vi "Update distance annotations.vi"(5 "Y axis max":dbl, 7 "Y axis min":dbl, 8 "error in (no error)":errorcluster, 9 "Anott. for update array in":i32[](array[numeric]), 10 "All cursors' dist.":T2, 11 "XY Graph":refnum<vi>) -> (0 "error out":errorcluster)   [LabVIEW 2014]
uses:
  Controls/dist. between cursors.ctl
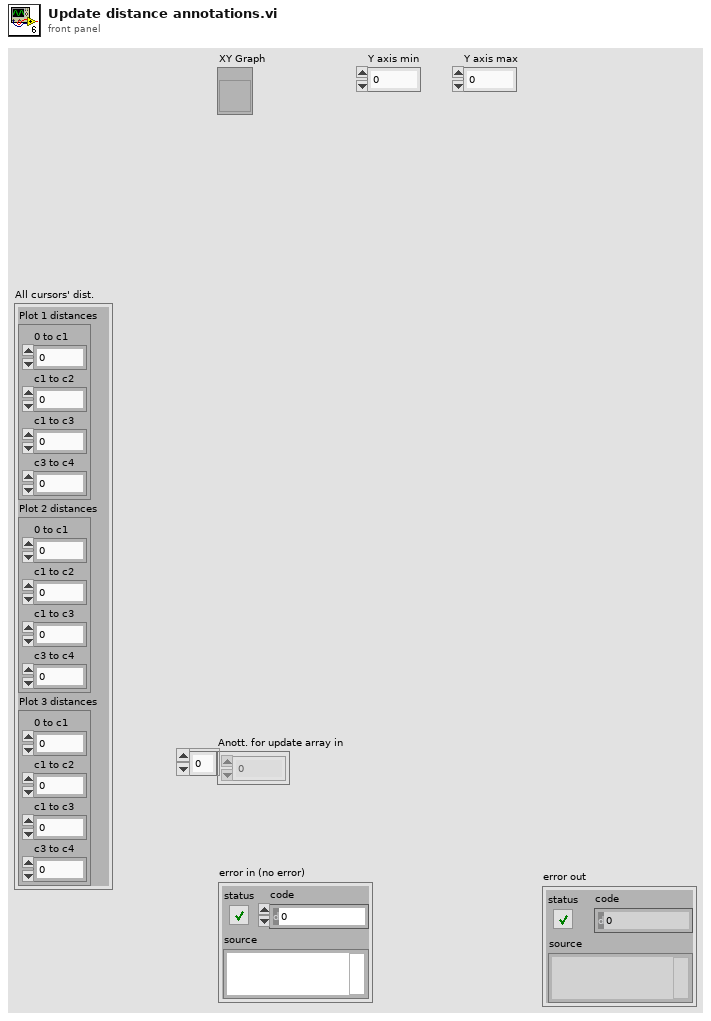
[diagram p1: front panel]
types:
  T1 = typedef "dist. between cursors.ctl" = cluster{"0 to c1":dbl, "c1 to c2":dbl, "c1 to c3":dbl, "c3 to c4":dbl}
  T2 = cluster{"Plot 1 distances":T1, "Plot 2 distances":T1, "Plot 3 distances":T1}
  T3 = enum16{"read", "write", "write number of cursors per plot only"}
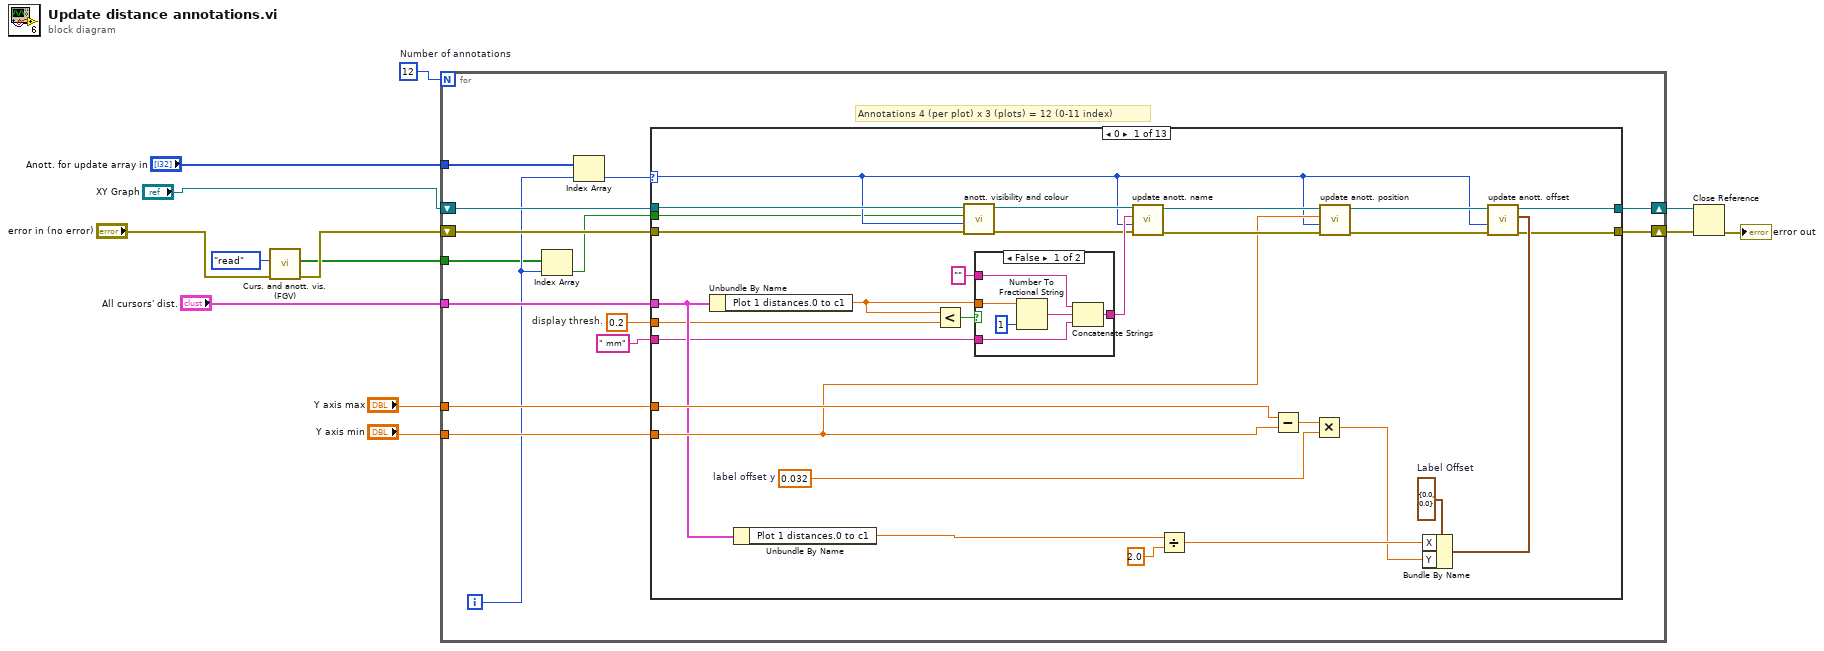
[diagram p0: block diagram]
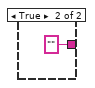
[diagram p2: hidden frame]
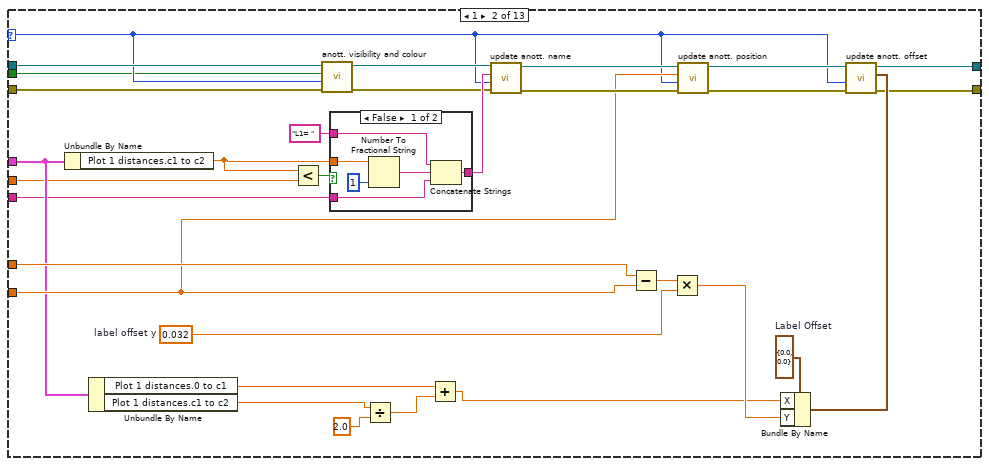
[diagram p3: hidden frame]
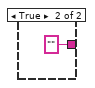
[diagram p4: hidden frame]
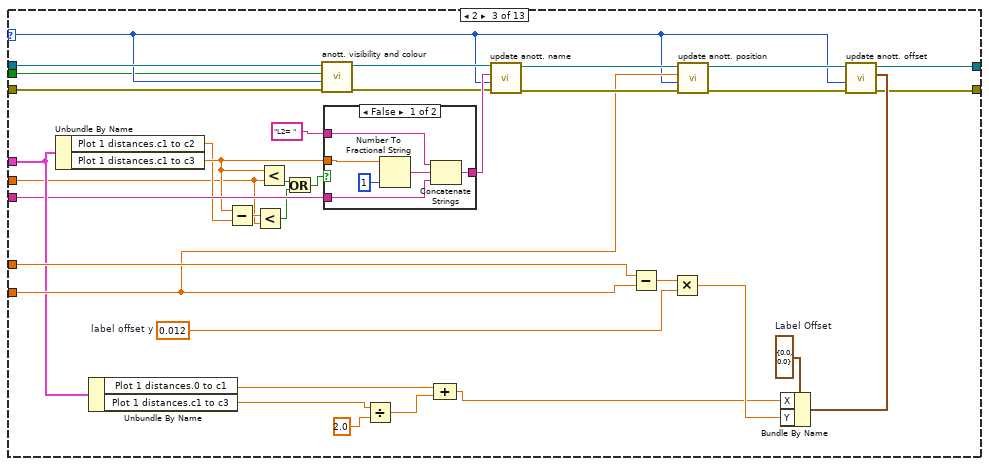
[diagram p5: hidden frame]
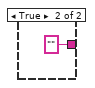
[diagram p6: hidden frame]
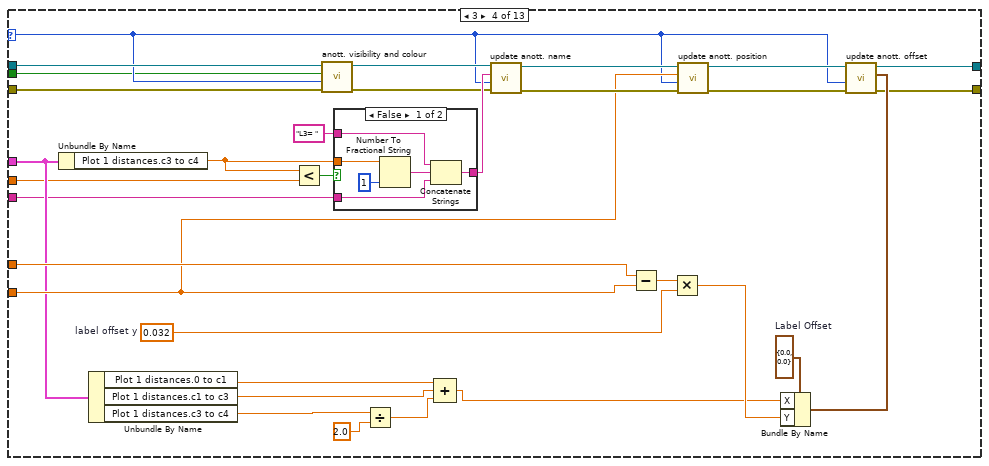
[diagram p7: hidden frame]
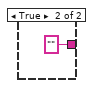
[diagram p8: hidden frame]
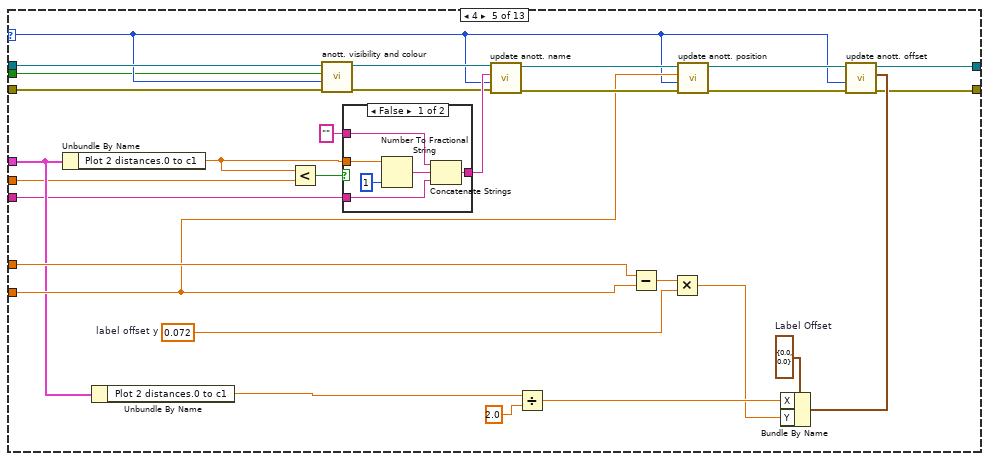
[diagram p9: hidden frame]
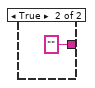
[diagram p10: hidden frame]
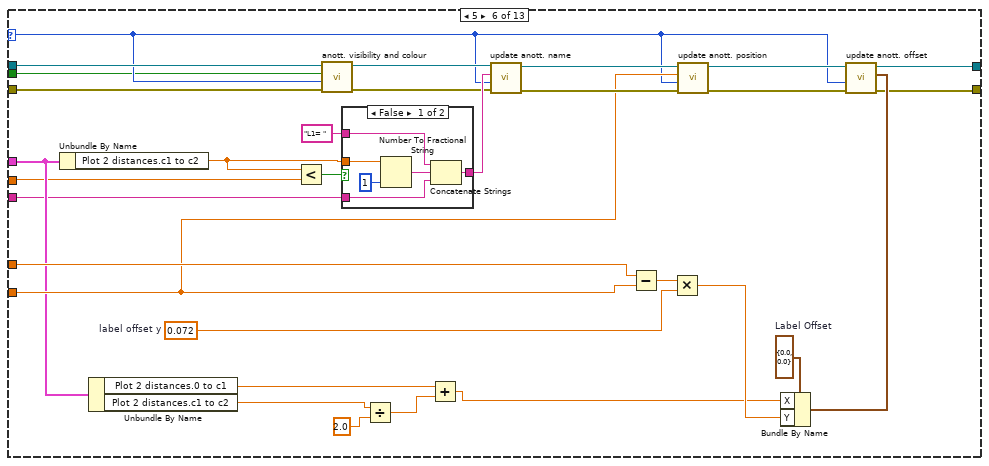
[diagram p11: hidden frame]
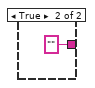
[diagram p12: hidden frame]
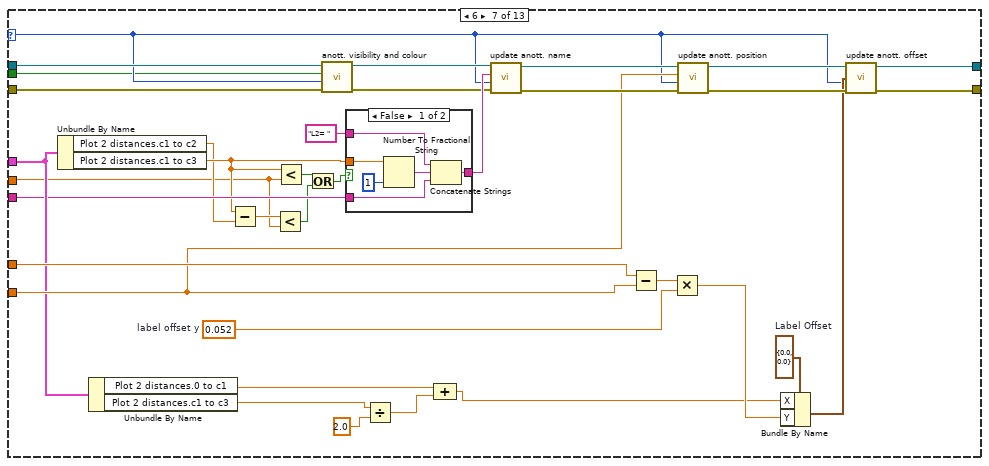
[diagram p13: hidden frame]
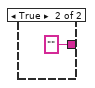
[diagram p14: hidden frame]
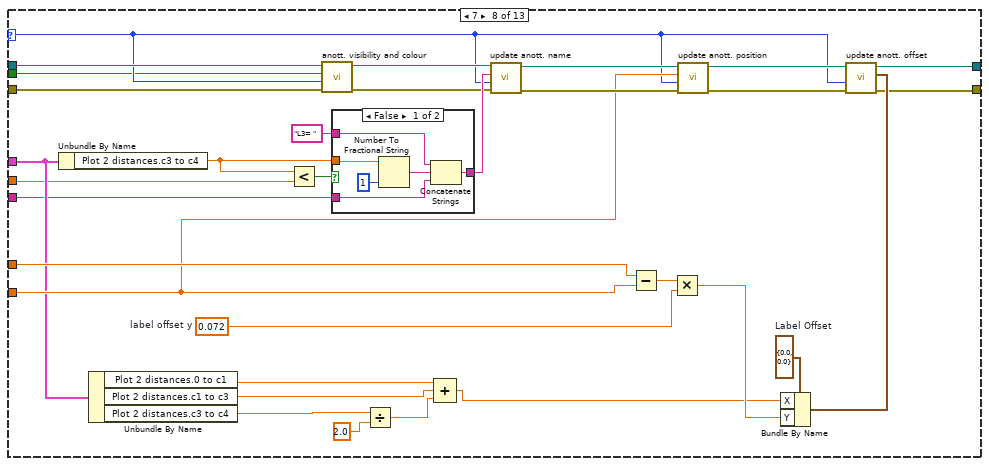
[diagram p15: hidden frame]
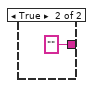
[diagram p16: hidden frame]
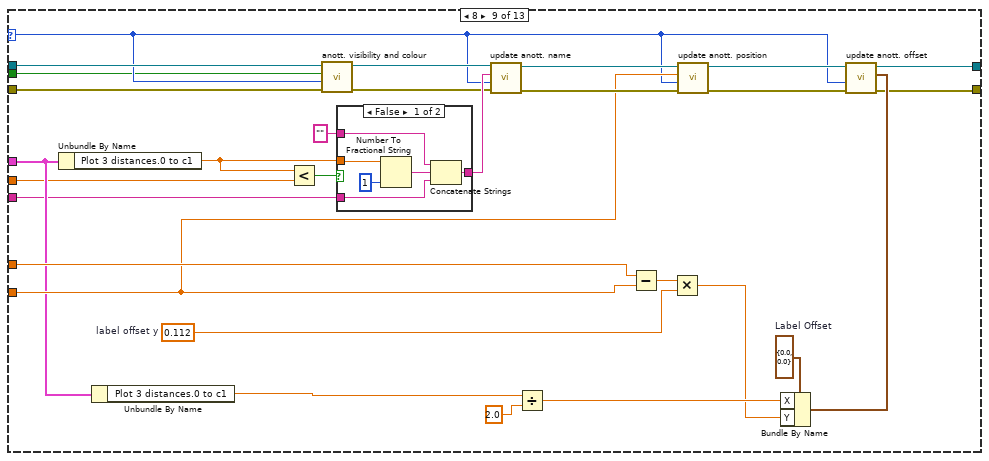
[diagram p17: hidden frame]
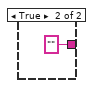
[diagram p18: hidden frame]
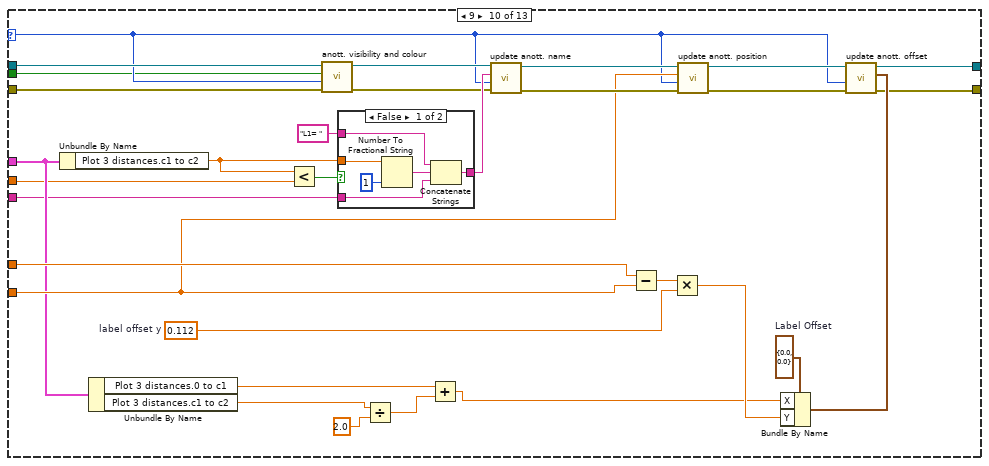
[diagram p19: hidden frame]
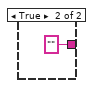
[diagram p20: hidden frame]
diagram:
  w7 = 12  # Number of annotations
  n1 = call "Curs. and anott. vis. (FGV).vi"("error in (no error)"="error in (no error)", "Enum"=T3."read") -> ("error out"=w5:errorcluster, "anott. visibility array out"=w3:bool[])  [unwired: 7 in, 1 out]
  n2 = for {
    N: w7 -> [_]
    tunnel: "Y axis max" -> [w27]
    tunnel: "Y axis min" -> [w26]
    tunnel: "All cursors' dist." -> [w21]
    shift-right: [w23] -> w10
    shift-left: w5 -> [w25]
    shift-right: [w22] -> w9
    shift-left: "XY Graph" -> [w24]
    tunnel: "Anott. for update array in" -> [w19]
    tunnel: w3 -> [w17]
    i -> [w18]
    w14 = 0.2  # display thresh.
    # "Annotations 4 (per plot) x 3 (plots) = 12 (0-11 index)"
    n3 = Index Array(array=w17, index=w18) -> (element=w16:bool)
    n4 = Index Array(array=w19, index=w18) -> (element=w20:i32)
    n5 = case shown="0" w20 {
      selector: w20 -> [w34 w71 w113 w154 w189 w226 w268 w309 w344 w381 w423 w464 _]
      tunnel: w27 -> [w56 w94 w136 w175 w211 w249 w291 w330 w366 w404 w446 w485 _]
      tunnel: w26 -> [w48 w88 w130 w169 w203 w243 w285 w324 w358 w398 w440 w479 _]
      tunnel: w25 -> [w42 w82 w124 w163 w197 w237 w279 w318 w352 w392 w434 w473 w493]
      tunnel: w24 -> [w40 w80 w122 w161 w195 w235 w277 w316 w350 w390 w432 w471 w494]
      tunnel: w21 -> [w39 w79 w121 w160 w194 w234 w276 w315 w349 w389 w431 w470 _]
      tunnel: [w37 w77 w119 w158 w192 w232 w274 w313 w347 w387 w429 w468 w493] -> w23
      tunnel: [w36 w76 w118 w157 w191 w231 w273 w312 w346 w386 w428 w467 w494] -> w22
      tunnel: w16 -> [w33 w69 w111 w149 w188 w224 w266 w304 w343 w379 w421 w459 _]
      tunnel: " mm" ("string") -> [w32 w68 w110 w148 w187 w223 w265 w303 w342 w378 w420 w458 _]
      tunnel: w14 -> [w29 w66 w103 w147 w186 w222 w257 w302 w341 w377 w413 w457 _]
      frame 0 {
        w35 = 0.032  # label offset y
        w54 = cluster{"X":dbl, "Y":dbl} {"X"=0.0, "Y"=0.0}  # Label Offset
        n6 = Unbundle By Name(w39) -> ("Plot 1 distances.0 to c1"=w30:dbl)
        n7 = Unbundle By Name(w39) -> ("Plot 1 distances.0 to c1"=w53:dbl)
        n8 = Less?(x=w30, y=w29) -> (x < y?=w31:bool)
        n9 = call "anott. visibility and colour.vi"("error in (no error)"=w42, "Annotation No"=w34, "Name Visible"=w33, "XYGraph in"=w40) -> ("error out"=w43:errorcluster, "XYGraph out"=w41:refnum<vi>)  [unwired: 6 in]
        n10 = case shown="False" w31 {
          tunnel: [w60 ""] -> w47
          tunnel: w30 -> [w59 _]
          tunnel: "" ("string") -> [w58 _]
          tunnel: w32 -> [w57 _]
          frame False {
            n11 = Number To Fractional String(number=w59, precision (6)=i16 1) -> (F-format string=w62:string)  [unwired: 2 in]
            n12 = Concatenate Strings(w58, w62, w57) -> (w60:string)
          }
          frame True {
          }
        }
        n13 = call "update anott. name.vi"("error in (no error)"=w43, "Annotation No"=w34, "Name"=w47, "XYGraph in"=w41) -> ("error out"=w50:errorcluster, "XYGraph out"=w49:refnum<vi>)  [unwired: 6 in]
        n14 = Divide(x=w53, y=2.0) -> (x/y=w52:dbl)
        n15 = Subtract(x=w56, y=w48) -> (x-y=w55:dbl)
        n16 = Multiply(x=w55, y=w35) -> (x*y=w51:dbl)
        n17 = call "update anott. position.vi"("error in (no error)"=w50, "Annotation No"=w34, "y axis min."=w48, "XYGraph in"=w49) -> ("error out"=w45:errorcluster, "XYGraph out"=w46:refnum<vi>)  [unwired: 6 in]
        n18 = Bundle By Name(cluster=w54, "X"=w52, "Y"=w51) -> (w44:cluster{"X":dbl, "Y":dbl})
        n19 = call "update anott. offset.vi"("error in (no error)"=w45, "Annotation No"=w34, "Label Offset"=w44, "XYGraph in"=w46) -> ("error out"=w37:errorcluster, "XYGraph out"=w36:refnum<vi>)  [unwired: 6 in]
      }
      frame 1 {
        w70 = 0.032  # label offset y
        w92 = cluster{"X":dbl, "Y":dbl} {"X"=0.0, "Y"=0.0}  # Label Offset
        n20 = Unbundle By Name(w79) -> ("Plot 1 distances.c1 to c2"=w67:dbl)
        n21 = Unbundle By Name(w79) -> ("Plot 1 distances.0 to c1"=w74:dbl, "Plot 1 distances.c1 to c2"=w75:dbl)
        n22 = Less?(x=w67, y=w66) -> (x < y?=w65:bool)
        n23 = call "anott. visibility and colour.vi"("error in (no error)"=w82, "Annotation No"=w71, "Name Visible"=w69, "XYGraph in"=w80) -> ("error out"=w83:errorcluster, "XYGraph out"=w81:refnum<vi>)  [unwired: 6 in]
        n24 = case shown="False" w65 {
          tunnel: [w98 ""] -> w87
          tunnel: w67 -> [w97 _]
          tunnel: "L1= " ("string") -> [w96 _]
          tunnel: w68 -> [w95 _]
          frame False {
            n25 = Number To Fractional String(number=w97, precision (6)=i16 1) -> (F-format string=w100:string)  [unwired: 2 in]
            n26 = Concatenate Strings(w96, w100, w95) -> (w98:string)
          }
          frame True {
          }
        }
        n27 = Divide(x=w75, y=2.0) -> (x/y=w73:dbl)
        n28 = Add(x=w74, y=w73) -> (x+y=w72:dbl)
        n29 = call "update anott. name.vi"("error in (no error)"=w83, "Annotation No"=w71, "Name"=w87, "XYGraph in"=w81) -> ("error out"=w90:errorcluster, "XYGraph out"=w89:refnum<vi>)  [unwired: 6 in]
        n30 = Subtract(x=w94, y=w88) -> (x-y=w93:dbl)
        n31 = Multiply(x=w93, y=w70) -> (x*y=w91:dbl)
        n32 = call "update anott. position.vi"("error in (no error)"=w90, "Annotation No"=w71, "y axis min."=w88, "XYGraph in"=w89) -> ("error out"=w85:errorcluster, "XYGraph out"=w86:refnum<vi>)  [unwired: 6 in]
        n33 = Bundle By Name(cluster=w92, "X"=w72, "Y"=w91) -> (w84:cluster{"X":dbl, "Y":dbl})
        n34 = call "update anott. offset.vi"("error in (no error)"=w85, "Annotation No"=w71, "Label Offset"=w84, "XYGraph in"=w86) -> ("error out"=w77:errorcluster, "XYGraph out"=w76:refnum<vi>)  [unwired: 6 in]
      }
      frame 2 {
        w112 = 0.012  # label offset y
        w134 = cluster{"X":dbl, "Y":dbl} {"X"=0.0, "Y"=0.0}  # Label Offset
        n35 = Unbundle By Name(w121) -> ("Plot 1 distances.c1 to c2"=w104:dbl, "Plot 1 distances.c1 to c3"=w105:dbl)
        n36 = Unbundle By Name(w121) -> ("Plot 1 distances.0 to c1"=w116:dbl, "Plot 1 distances.c1 to c3"=w117:dbl)
        n37 = Subtract(x=w105, y=w104) -> (x-y=w106:dbl)
        n38 = Less?(x=w106, y=w103) -> (x < y?=w102:bool)
        n39 = Less?(x=w105, y=w103) -> (x < y?=w108:bool)
        n40 = Or(x=w108, y=w102) -> (x .or. y?=w107:bool)
        n41 = call "anott. visibility and colour.vi"("error in (no error)"=w124, "Annotation No"=w113, "Name Visible"=w111, "XYGraph in"=w122) -> ("error out"=w125:errorcluster, "XYGraph out"=w123:refnum<vi>)  [unwired: 6 in]
        n42 = case shown="False" w107 {
          tunnel: [w140 ""] -> w129
          tunnel: w105 -> [w139 _]
          tunnel: "L2= " ("string") -> [w138 _]
          tunnel: w110 -> [w137 _]
          frame False {
            n43 = Number To Fractional String(number=w139, precision (6)=i16 1) -> (F-format string=w142:string)  [unwired: 2 in]
            n44 = Concatenate Strings(w138, w142, w137) -> (w140:string)
          }
          frame True {
          }
        }
        n45 = Divide(x=w117, y=2.0) -> (x/y=w115:dbl)
        n46 = Compound Arithmetic op=ADD(w116, w115) -> (w114:dbl)
        n47 = call "update anott. name.vi"("error in (no error)"=w125, "Annotation No"=w113, "Name"=w129, "XYGraph in"=w123) -> ("error out"=w132:errorcluster, "XYGraph out"=w131:refnum<vi>)  [unwired: 6 in]
        n48 = Subtract(x=w136, y=w130) -> (x-y=w135:dbl)
        n49 = Multiply(x=w135, y=w112) -> (x*y=w133:dbl)
        n50 = call "update anott. position.vi"("error in (no error)"=w132, "Annotation No"=w113, "y axis min."=w130, "XYGraph in"=w131) -> ("error out"=w127:errorcluster, "XYGraph out"=w128:refnum<vi>)  [unwired: 6 in]
        n51 = Bundle By Name(cluster=w134, "X"=w114, "Y"=w133) -> (w126:cluster{"X":dbl, "Y":dbl})
        n52 = call "update anott. offset.vi"("error in (no error)"=w127, "Annotation No"=w113, "Label Offset"=w126, "XYGraph in"=w128) -> ("error out"=w119:errorcluster, "XYGraph out"=w118:refnum<vi>)  [unwired: 6 in]
      }
      frame 3 {
        w150 = 0.032  # label offset y
        w173 = cluster{"X":dbl, "Y":dbl} {"X"=0.0, "Y"=0.0}  # Label Offset
        n53 = Unbundle By Name(w160) -> ("Plot 1 distances.c3 to c4"=w146:dbl)
        n54 = Unbundle By Name(w160) -> ("Plot 1 distances.0 to c1"=w156:dbl, "Plot 1 distances.c1 to c3"=w151:dbl, "Plot 1 distances.c3 to c4"=w153:dbl)
        n55 = Less?(x=w146, y=w147) -> (x < y?=w145:bool)
        n56 = call "anott. visibility and colour.vi"("error in (no error)"=w163, "Annotation No"=w154, "Name Visible"=w149, "XYGraph in"=w161) -> ("error out"=w164:errorcluster, "XYGraph out"=w162:refnum<vi>)  [unwired: 6 in]
        n57 = case shown="False" w145 {
          tunnel: [w179 ""] -> w168
          tunnel: w146 -> [w178 _]
          tunnel: "L3= " ("string") -> [w177 _]
          tunnel: w148 -> [w176 _]
          frame False {
            n58 = Number To Fractional String(number=w178, precision (6)=i16 1) -> (F-format string=w181:string)  [unwired: 2 in]
            n59 = Concatenate Strings(w177, w181, w176) -> (w179:string)
          }
          frame True {
          }
        }
        n60 = Divide(x=w153, y=2.0) -> (x/y=w152:dbl)
        n61 = Compound Arithmetic op=ADD(w156, w151, w152) -> (w155:dbl)
        n62 = call "update anott. name.vi"("error in (no error)"=w164, "Annotation No"=w154, "Name"=w168, "XYGraph in"=w162) -> ("error out"=w171:errorcluster, "XYGraph out"=w170:refnum<vi>)  [unwired: 6 in]
        n63 = Subtract(x=w175, y=w169) -> (x-y=w174:dbl)
        n64 = Multiply(x=w174, y=w150) -> (x*y=w172:dbl)
        n65 = call "update anott. position.vi"("error in (no error)"=w171, "Annotation No"=w154, "y axis min."=w169, "XYGraph in"=w170) -> ("error out"=w166:errorcluster, "XYGraph out"=w167:refnum<vi>)  [unwired: 6 in]
        n66 = Bundle By Name(cluster=w173, "X"=w155, "Y"=w172) -> (w165:cluster{"X":dbl, "Y":dbl})
        n67 = call "update anott. offset.vi"("error in (no error)"=w166, "Annotation No"=w154, "Label Offset"=w165, "XYGraph in"=w167) -> ("error out"=w158:errorcluster, "XYGraph out"=w157:refnum<vi>)  [unwired: 6 in]
      }
      frame 4 {
        w190 = 0.072  # label offset y
        w209 = cluster{"X":dbl, "Y":dbl} {"X"=0.0, "Y"=0.0}  # Label Offset
        n68 = Unbundle By Name(w194) -> ("Plot 2 distances.0 to c1"=w185:dbl)
        n69 = Unbundle By Name(w194) -> ("Plot 2 distances.0 to c1"=w208:dbl)
        n70 = Less?(x=w185, y=w186) -> (x < y?=w184:bool)
        n71 = call "anott. visibility and colour.vi"("error in (no error)"=w197, "Annotation No"=w189, "Name Visible"=w188, "XYGraph in"=w195) -> ("error out"=w198:errorcluster, "XYGraph out"=w196:refnum<vi>)  [unwired: 6 in]
        n72 = case shown="False" w184 {
          tunnel: [w215 ""] -> w202
          tunnel: w185 -> [w214 _]
          tunnel: "" ("string") -> [w213 _]
          tunnel: w187 -> [w212 _]
          frame False {
            n73 = Number To Fractional String(number=w214, precision (6)=i16 1) -> (F-format string=w217:string)  [unwired: 2 in]
            n74 = Concatenate Strings(w213, w217, w212) -> (w215:string)
          }
          frame True {
          }
        }
        n75 = call "update anott. name.vi"("error in (no error)"=w198, "Annotation No"=w189, "Name"=w202, "XYGraph in"=w196) -> ("error out"=w205:errorcluster, "XYGraph out"=w204:refnum<vi>)  [unwired: 6 in]
        n76 = Divide(x=w208, y=2.0) -> (x/y=w207:dbl)
        n77 = Subtract(x=w211, y=w203) -> (x-y=w210:dbl)
        n78 = Multiply(x=w210, y=w190) -> (x*y=w206:dbl)
        n79 = call "update anott. position.vi"("error in (no error)"=w205, "Annotation No"=w189, "y axis min."=w203, "XYGraph in"=w204) -> ("error out"=w200:errorcluster, "XYGraph out"=w201:refnum<vi>)  [unwired: 6 in]
        n80 = Bundle By Name(cluster=w209, "X"=w207, "Y"=w206) -> (w199:cluster{"X":dbl, "Y":dbl})
        n81 = call "update anott. offset.vi"("error in (no error)"=w200, "Annotation No"=w189, "Label Offset"=w199, "XYGraph in"=w201) -> ("error out"=w192:errorcluster, "XYGraph out"=w191:refnum<vi>)  [unwired: 6 in]
      }
      frame 5 {
        w225 = 0.072  # label offset y
        w247 = cluster{"X":dbl, "Y":dbl} {"X"=0.0, "Y"=0.0}  # Label Offset
        n82 = Unbundle By Name(w234) -> ("Plot 2 distances.c1 to c2"=w221:dbl)
        n83 = Unbundle By Name(w234) -> ("Plot 2 distances.0 to c1"=w229:dbl, "Plot 2 distances.c1 to c2"=w230:dbl)
        n84 = Less?(x=w221, y=w222) -> (x < y?=w220:bool)
        n85 = call "anott. visibility and colour.vi"("error in (no error)"=w237, "Annotation No"=w226, "Name Visible"=w224, "XYGraph in"=w235) -> ("error out"=w238:errorcluster, "XYGraph out"=w236:refnum<vi>)  [unwired: 6 in]
        n86 = case shown="False" w220 {
          tunnel: [w253 ""] -> w242
          tunnel: w221 -> [w252 _]
          tunnel: "L1= " ("string") -> [w251 _]
          tunnel: w223 -> [w250 _]
          frame False {
            n87 = Number To Fractional String(number=w252, precision (6)=i16 1) -> (F-format string=w255:string)  [unwired: 2 in]
            n88 = Concatenate Strings(w251, w255, w250) -> (w253:string)
          }
          frame True {
          }
        }
        n89 = Divide(x=w230, y=2.0) -> (x/y=w228:dbl)
        n90 = Add(x=w229, y=w228) -> (x+y=w227:dbl)
        n91 = call "update anott. name.vi"("error in (no error)"=w238, "Annotation No"=w226, "Name"=w242, "XYGraph in"=w236) -> ("error out"=w245:errorcluster, "XYGraph out"=w244:refnum<vi>)  [unwired: 6 in]
        n92 = Subtract(x=w249, y=w243) -> (x-y=w248:dbl)
        n93 = Multiply(x=w248, y=w225) -> (x*y=w246:dbl)
        n94 = call "update anott. position.vi"("error in (no error)"=w245, "Annotation No"=w226, "y axis min."=w243, "XYGraph in"=w244) -> ("error out"=w240:errorcluster, "XYGraph out"=w241:refnum<vi>)  [unwired: 6 in]
        n95 = Bundle By Name(cluster=w247, "X"=w227, "Y"=w246) -> (w239:cluster{"X":dbl, "Y":dbl})
        n96 = call "update anott. offset.vi"("error in (no error)"=w240, "Annotation No"=w226, "Label Offset"=w239, "XYGraph in"=w241) -> ("error out"=w232:errorcluster, "XYGraph out"=w231:refnum<vi>)  [unwired: 6 in]
      }
      frame 6 {
        w267 = 0.052  # label offset y
        w289 = cluster{"X":dbl, "Y":dbl} {"X"=0.0, "Y"=0.0}  # Label Offset
        n97 = Unbundle By Name(w276) -> ("Plot 2 distances.c1 to c2"=w259:dbl, "Plot 2 distances.c1 to c3"=w260:dbl)
        n98 = Unbundle By Name(w276) -> ("Plot 2 distances.0 to c1"=w271:dbl, "Plot 2 distances.c1 to c3"=w272:dbl)
        n99 = Subtract(x=w260, y=w259) -> (x-y=w258:dbl)
        n100 = Less?(x=w258, y=w257) -> (x < y?=w261:bool)
        n101 = Less?(x=w260, y=w257) -> (x < y?=w262:bool)
        n102 = Or(x=w262, y=w261) -> (x .or. y?=w263:bool)
        n103 = call "anott. visibility and colour.vi"("error in (no error)"=w279, "Annotation No"=w268, "Name Visible"=w266, "XYGraph in"=w277) -> ("error out"=w280:errorcluster, "XYGraph out"=w278:refnum<vi>)  [unwired: 6 in]
        n104 = case shown="False" w263 {
          tunnel: [w295 ""] -> w284
          tunnel: w260 -> [w294 _]
          tunnel: "L2= " ("string") -> [w293 _]
          tunnel: w265 -> [w292 _]
          frame False {
            n105 = Number To Fractional String(number=w294, precision (6)=i16 1) -> (F-format string=w297:string)  [unwired: 2 in]
            n106 = Concatenate Strings(w293, w297, w292) -> (w295:string)
          }
          frame True {
          }
        }
        n107 = Divide(x=w272, y=2.0) -> (x/y=w270:dbl)
        n108 = Compound Arithmetic op=ADD(w271, w270) -> (w269:dbl)
        n109 = call "update anott. name.vi"("error in (no error)"=w280, "Annotation No"=w268, "Name"=w284, "XYGraph in"=w278) -> ("error out"=w287:errorcluster, "XYGraph out"=w286:refnum<vi>)  [unwired: 6 in]
        n110 = Subtract(x=w291, y=w285) -> (x-y=w290:dbl)
        n111 = Multiply(x=w290, y=w267) -> (x*y=w288:dbl)
        n112 = call "update anott. position.vi"("error in (no error)"=w287, "Annotation No"=w268, "y axis min."=w285, "XYGraph in"=w286) -> ("error out"=w282:errorcluster, "XYGraph out"=w283:refnum<vi>)  [unwired: 6 in]
        n113 = Bundle By Name(cluster=w289, "X"=w269, "Y"=w288) -> (w281:cluster{"X":dbl, "Y":dbl})
        n114 = call "update anott. offset.vi"("error in (no error)"=w282, "Annotation No"=w268, "Label Offset"=w281, "XYGraph in"=w283) -> ("error out"=w274:errorcluster, "XYGraph out"=w273:refnum<vi>)  [unwired: 6 in]
      }
      frame 7 {
        w305 = 0.072  # label offset y
        w328 = cluster{"X":dbl, "Y":dbl} {"X"=0.0, "Y"=0.0}  # Label Offset
        n115 = Unbundle By Name(w315) -> ("Plot 2 distances.c3 to c4"=w301:dbl)
        n116 = Unbundle By Name(w315) -> ("Plot 2 distances.0 to c1"=w311:dbl, "Plot 2 distances.c1 to c3"=w306:dbl, "Plot 2 distances.c3 to c4"=w308:dbl)
        n117 = Less?(x=w301, y=w302) -> (x < y?=w300:bool)
        n118 = call "anott. visibility and colour.vi"("error in (no error)"=w318, "Annotation No"=w309, "Name Visible"=w304, "XYGraph in"=w316) -> ("error out"=w319:errorcluster, "XYGraph out"=w317:refnum<vi>)  [unwired: 6 in]
        n119 = case shown="False" w300 {
          tunnel: [w334 ""] -> w323
          tunnel: w301 -> [w333 _]
          tunnel: "L3= " ("string") -> [w332 _]
          tunnel: w303 -> [w331 _]
          frame False {
            n120 = Number To Fractional String(number=w333, precision (6)=i16 1) -> (F-format string=w336:string)  [unwired: 2 in]
            n121 = Concatenate Strings(w332, w336, w331) -> (w334:string)
          }
          frame True {
          }
        }
        n122 = Divide(x=w308, y=2.0) -> (x/y=w307:dbl)
        n123 = Compound Arithmetic op=ADD(w311, w306, w307) -> (w310:dbl)
        n124 = call "update anott. name.vi"("error in (no error)"=w319, "Annotation No"=w309, "Name"=w323, "XYGraph in"=w317) -> ("error out"=w326:errorcluster, "XYGraph out"=w325:refnum<vi>)  [unwired: 6 in]
        n125 = Subtract(x=w330, y=w324) -> (x-y=w329:dbl)
        n126 = Multiply(x=w329, y=w305) -> (x*y=w327:dbl)
        n127 = call "update anott. position.vi"("error in (no error)"=w326, "Annotation No"=w309, "y axis min."=w324, "XYGraph in"=w325) -> ("error out"=w321:errorcluster, "XYGraph out"=w322:refnum<vi>)  [unwired: 6 in]
        n128 = Bundle By Name(cluster=w328, "X"=w310, "Y"=w327) -> (w320:cluster{"X":dbl, "Y":dbl})
        n129 = call "update anott. offset.vi"("error in (no error)"=w321, "Annotation No"=w309, "Label Offset"=w320, "XYGraph in"=w322) -> ("error out"=w313:errorcluster, "XYGraph out"=w312:refnum<vi>)  [unwired: 6 in]
      }
      frame 8 {
        w345 = 0.112  # label offset y
        w364 = cluster{"X":dbl, "Y":dbl} {"X"=0.0, "Y"=0.0}  # Label Offset
        n130 = Unbundle By Name(w349) -> ("Plot 3 distances.0 to c1"=w340:dbl)
        n131 = Unbundle By Name(w349) -> ("Plot 3 distances.0 to c1"=w363:dbl)
        n132 = Less?(x=w340, y=w341) -> (x < y?=w339:bool)
        n133 = call "anott. visibility and colour.vi"("error in (no error)"=w352, "Annotation No"=w344, "Name Visible"=w343, "XYGraph in"=w350) -> ("error out"=w353:errorcluster, "XYGraph out"=w351:refnum<vi>)  [unwired: 6 in]
        n134 = case shown="False" w339 {
          tunnel: [w370 ""] -> w357
          tunnel: w340 -> [w369 _]
          tunnel: "" ("string") -> [w368 _]
          tunnel: w342 -> [w367 _]
          frame False {
            n135 = Number To Fractional String(number=w369, precision (6)=i16 1) -> (F-format string=w372:string)  [unwired: 2 in]
            n136 = Concatenate Strings(w368, w372, w367) -> (w370:string)
          }
          frame True {
          }
        }
        n137 = call "update anott. name.vi"("error in (no error)"=w353, "Annotation No"=w344, "Name"=w357, "XYGraph in"=w351) -> ("error out"=w360:errorcluster, "XYGraph out"=w359:refnum<vi>)  [unwired: 6 in]
        n138 = Divide(x=w363, y=2.0) -> (x/y=w362:dbl)
        n139 = Subtract(x=w366, y=w358) -> (x-y=w365:dbl)
        n140 = Multiply(x=w365, y=w345) -> (x*y=w361:dbl)
        n141 = call "update anott. position.vi"("error in (no error)"=w360, "Annotation No"=w344, "y axis min."=w358, "XYGraph in"=w359) -> ("error out"=w355:errorcluster, "XYGraph out"=w356:refnum<vi>)  [unwired: 6 in]
        n142 = Bundle By Name(cluster=w364, "X"=w362, "Y"=w361) -> (w354:cluster{"X":dbl, "Y":dbl})
        n143 = call "update anott. offset.vi"("error in (no error)"=w355, "Annotation No"=w344, "Label Offset"=w354, "XYGraph in"=w356) -> ("error out"=w347:errorcluster, "XYGraph out"=w346:refnum<vi>)  [unwired: 6 in]
      }
      frame 9 {
        w380 = 0.112  # label offset y
        w402 = cluster{"X":dbl, "Y":dbl} {"X"=0.0, "Y"=0.0}  # Label Offset
        n144 = Unbundle By Name(w389) -> ("Plot 3 distances.c1 to c2"=w376:dbl)
        n145 = Unbundle By Name(w389) -> ("Plot 3 distances.0 to c1"=w384:dbl, "Plot 3 distances.c1 to c2"=w385:dbl)
        n146 = Less?(x=w376, y=w377) -> (x < y?=w375:bool)
        n147 = call "anott. visibility and colour.vi"("error in (no error)"=w392, "Annotation No"=w381, "Name Visible"=w379, "XYGraph in"=w390) -> ("error out"=w393:errorcluster, "XYGraph out"=w391:refnum<vi>)  [unwired: 6 in]
        n148 = case shown="False" w375 {
          tunnel: [w408 ""] -> w397
          tunnel: w376 -> [w407 _]
          tunnel: "L1= " ("string") -> [w406 _]
          tunnel: w378 -> [w405 _]
          frame False {
            n149 = Number To Fractional String(number=w407, precision (6)=i16 1) -> (F-format string=w410:string)  [unwired: 2 in]
            n150 = Concatenate Strings(w406, w410, w405) -> (w408:string)
          }
          frame True {
          }
        }
        n151 = Divide(x=w385, y=2.0) -> (x/y=w383:dbl)
        n152 = Add(x=w384, y=w383) -> (x+y=w382:dbl)
        n153 = call "update anott. name.vi"("error in (no error)"=w393, "Annotation No"=w381, "Name"=w397, "XYGraph in"=w391) -> ("error out"=w400:errorcluster, "XYGraph out"=w399:refnum<vi>)  [unwired: 6 in]
        n154 = Subtract(x=w404, y=w398) -> (x-y=w403:dbl)
        n155 = Multiply(x=w403, y=w380) -> (x*y=w401:dbl)
        n156 = call "update anott. position.vi"("error in (no error)"=w400, "Annotation No"=w381, "y axis min."=w398, "XYGraph in"=w399) -> ("error out"=w395:errorcluster, "XYGraph out"=w396:refnum<vi>)  [unwired: 6 in]
        n157 = Bundle By Name(cluster=w402, "X"=w382, "Y"=w401) -> (w394:cluster{"X":dbl, "Y":dbl})
        n158 = call "update anott. offset.vi"("error in (no error)"=w395, "Annotation No"=w381, "Label Offset"=w394, "XYGraph in"=w396) -> ("error out"=w387:errorcluster, "XYGraph out"=w386:refnum<vi>)  [unwired: 6 in]
      }
      frame 10 {
        w422 = 0.092  # label offset y
        w444 = cluster{"X":dbl, "Y":dbl} {"X"=0.0, "Y"=0.0}  # Label Offset
        n159 = Unbundle By Name(w431) -> ("Plot 3 distances.c1 to c2"=w417:dbl, "Plot 3 distances.c1 to c3"=w418:dbl)
        n160 = Unbundle By Name(w431) -> ("Plot 3 distances.0 to c1"=w426:dbl, "Plot 3 distances.c1 to c3"=w427:dbl)
        n161 = Subtract(x=w418, y=w417) -> (x-y=w414:dbl)
        n162 = Less?(x=w418, y=w413) -> (x < y?=w416:bool)
        n163 = Less?(x=w414, y=w413) -> (x < y?=w412:bool)
        n164 = Or(x=w416, y=w412) -> (x .or. y?=w415:bool)
        n165 = call "anott. visibility and colour.vi"("error in (no error)"=w434, "Annotation No"=w423, "Name Visible"=w421, "XYGraph in"=w432) -> ("error out"=w435:errorcluster, "XYGraph out"=w433:refnum<vi>)  [unwired: 6 in]
        n166 = case shown="False" w415 {
          tunnel: [w450 ""] -> w439
          tunnel: w418 -> [w449 _]
          tunnel: "L2= " ("string") -> [w448 _]
          tunnel: w420 -> [w447 _]
          frame False {
            n167 = Number To Fractional String(number=w449, precision (6)=i16 1) -> (F-format string=w452:string)  [unwired: 2 in]
            n168 = Concatenate Strings(w448, w452, w447) -> (w450:string)
          }
          frame True {
          }
        }
        n169 = Divide(x=w427, y=2.0) -> (x/y=w425:dbl)
        n170 = Compound Arithmetic op=ADD(w426, w425) -> (w424:dbl)
        n171 = call "update anott. name.vi"("error in (no error)"=w435, "Annotation No"=w423, "Name"=w439, "XYGraph in"=w433) -> ("error out"=w442:errorcluster, "XYGraph out"=w441:refnum<vi>)  [unwired: 6 in]
        n172 = Subtract(x=w446, y=w440) -> (x-y=w445:dbl)
        n173 = Multiply(x=w445, y=w422) -> (x*y=w443:dbl)
        n174 = call "update anott. position.vi"("error in (no error)"=w442, "Annotation No"=w423, "y axis min."=w440, "XYGraph in"=w441) -> ("error out"=w437:errorcluster, "XYGraph out"=w438:refnum<vi>)  [unwired: 6 in]
        n175 = Bundle By Name(cluster=w444, "X"=w424, "Y"=w443) -> (w436:cluster{"X":dbl, "Y":dbl})
        n176 = call "update anott. offset.vi"("error in (no error)"=w437, "Annotation No"=w423, "Label Offset"=w436, "XYGraph in"=w438) -> ("error out"=w429:errorcluster, "XYGraph out"=w428:refnum<vi>)  [unwired: 6 in]
      }
      frame 11 {
        w460 = 0.112  # label offset y
        w483 = cluster{"X":dbl, "Y":dbl} {"X"=0.0, "Y"=0.0}  # Label Offset
        n177 = Unbundle By Name(w470) -> ("Plot 3 distances.c3 to c4"=w456:dbl)
        n178 = Unbundle By Name(w470) -> ("Plot 3 distances.0 to c1"=w466:dbl, "Plot 3 distances.c1 to c3"=w461:dbl, "Plot 3 distances.c3 to c4"=w463:dbl)
        n179 = Less?(x=w456, y=w457) -> (x < y?=w455:bool)
        n180 = call "anott. visibility and colour.vi"("error in (no error)"=w473, "Annotation No"=w464, "Name Visible"=w459, "XYGraph in"=w471) -> ("error out"=w474:errorcluster, "XYGraph out"=w472:refnum<vi>)  [unwired: 6 in]
        n181 = case shown="False" w455 {
          tunnel: [w489 ""] -> w478
          tunnel: w456 -> [w488 _]
          tunnel: "L3= " ("string") -> [w487 _]
          tunnel: w458 -> [w486 _]
          frame False {
            n182 = Number To Fractional String(number=w488, precision (6)=i16 1) -> (F-format string=w491:string)  [unwired: 2 in]
            n183 = Concatenate Strings(w487, w491, w486) -> (w489:string)
          }
          frame True {
          }
        }
        n184 = Divide(x=w463, y=2.0) -> (x/y=w462:dbl)
        n185 = Compound Arithmetic op=ADD(w466, w461, w462) -> (w465:dbl)
        n186 = call "update anott. name.vi"("error in (no error)"=w474, "Annotation No"=w464, "Name"=w478, "XYGraph in"=w472) -> ("error out"=w481:errorcluster, "XYGraph out"=w480:refnum<vi>)  [unwired: 6 in]
        n187 = Subtract(x=w485, y=w479) -> (x-y=w484:dbl)
        n188 = Multiply(x=w484, y=w460) -> (x*y=w482:dbl)
        n189 = call "update anott. position.vi"("error in (no error)"=w481, "Annotation No"=w464, "y axis min."=w479, "XYGraph in"=w480) -> ("error out"=w476:errorcluster, "XYGraph out"=w477:refnum<vi>)  [unwired: 6 in]
        n190 = Bundle By Name(cluster=w483, "X"=w465, "Y"=w482) -> (w475:cluster{"X":dbl, "Y":dbl})
        n191 = call "update anott. offset.vi"("error in (no error)"=w476, "Annotation No"=w464, "Label Offset"=w475, "XYGraph in"=w477) -> ("error out"=w468:errorcluster, "XYGraph out"=w467:refnum<vi>)  [unwired: 6 in]
      }
      frame 12, Default {
        # "Empty case to be use for anottation which are not to be updated (CPU usage reduction)"
      }
    }
  }
  n192 = Close Reference(reference=w9, error in (no error)=w10) -> (error out=→"error out":errorcluster)
